vi "Timestamp_Compare.vi"() -> ()   [LabVIEW 2020]
panel:
  out "Camera Timestamp (UTC)":u64[](array[numeric])
  out "Camera Source Timestamp (UTC)":u64[](array[numeric])
  out "ENET First Timestamp Delta Difference":dbl format="%#_9g"
  out "CAN First Timestamp Delta Difference":dbl format="%#_9g"
  out "Camera First Timestamp Delta Difference":dbl[](array[numeric]) format="%#_9g"
  out "CAN Source Timestamp Delta":dbl format="%#_9f"
  out "ENET Source First Timestamp Delta":dbl format="%#_9f"
  in  "ENET Source T0 Time Stamp":timestamp=timestamp(3758873246.099163 s since 1904-01-01) format="%<%.6X\n%x>T"
  out "ENET First Timestamp Delta":dbl format="%#_9f"
  out "CAN First Timestamp Delta":dbl format="%#_9f"
  in  "ENET Receive First Time":timestamp=timestamp(3762227548.6655436 s since 1904-01-01) format="%<%.6X\n%x>T"
  in  "CAN Receive First Time":timestamp=timestamp(3762227536.6965528 s since 1904-01-01) format="%<%.6X\n%x>T"
  in  "CAN Source First Frame Relative Timestamp (s)":dbl=73.619141 format="%#_9g"
  in  "CAN Source T0 Time Stamp":timestamp=timestamp(3758873160.511 s since 1904-01-01)
  out "Camera Source First Timestamp Delta":dbl[](array[numeric]) format="%#_9f"
  out "Camera First Timestamp Delta":dbl[](array[numeric]) format="%#_9f"
  in  "Timestamp Compare Base Index":i32
  in  "Camera T0 TDMS":timestamp=timestamp(3762227502.1926026 s since 1904-01-01) format="%<%.6X\n%x>T"
  in  "Camera Source Timestamp Txt Path":path[](array[path])=[path "E:/Xiaomi_Source/RDMA_FVC0/time.txt", path "E:/Xiaomi_Source/RDMA_side0/time.txt"]
  in  "Source Timestamp from txt File":bool=TRUE
  out "error out":errorcluster
  in  "Camera Timestamp TDMS Path":path[](array[path])=[path "E:/Xiaomi_Test/4k_265_time.tdms", path "E:/Xiaomi_Test/2k_265_time.tdms"]
  in  "Skip First N Timestamp":i32=1
  in  "Camera Source_Timestamp (ns) type":T1(array[ring])
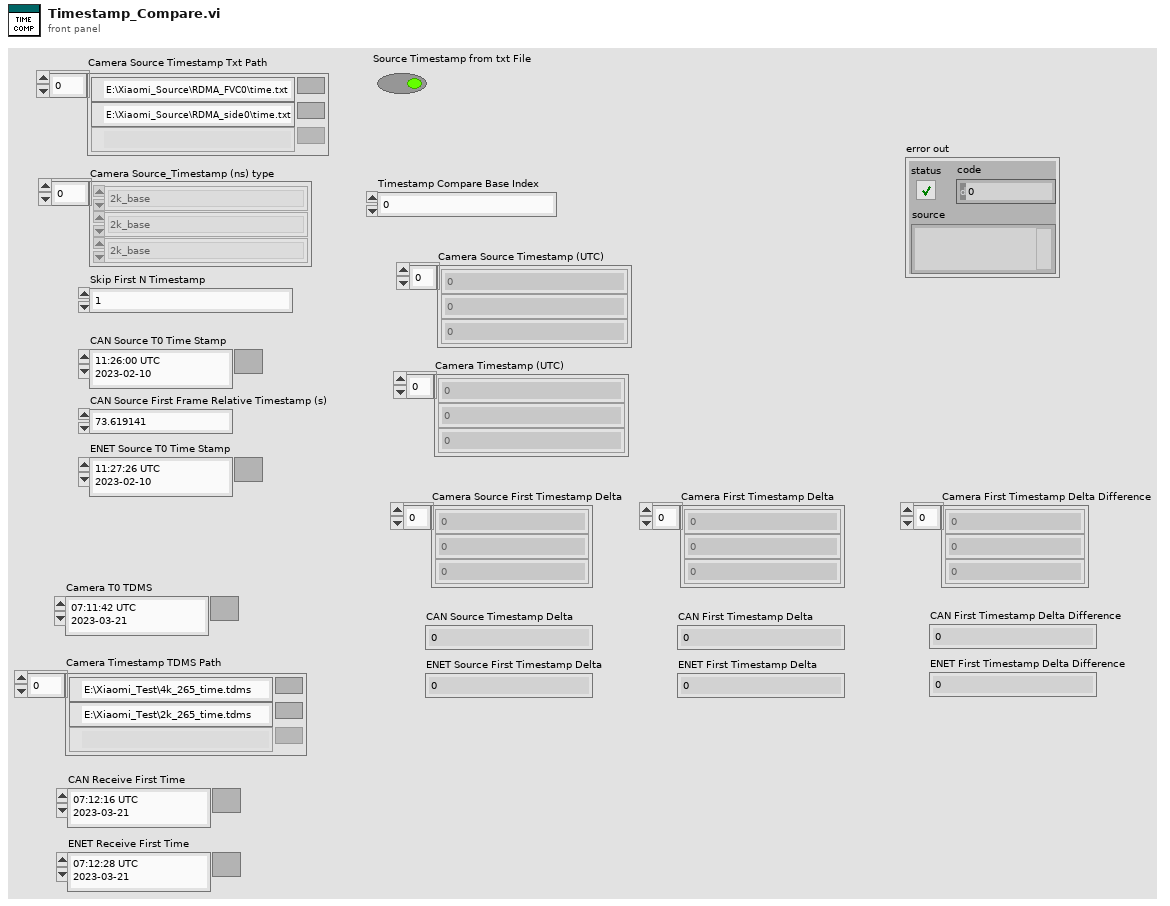
[diagram p1: front panel]
types:
  T1 = enum16{"2k_base", "2k_noise", "4k_base", "4k_noise"}[]
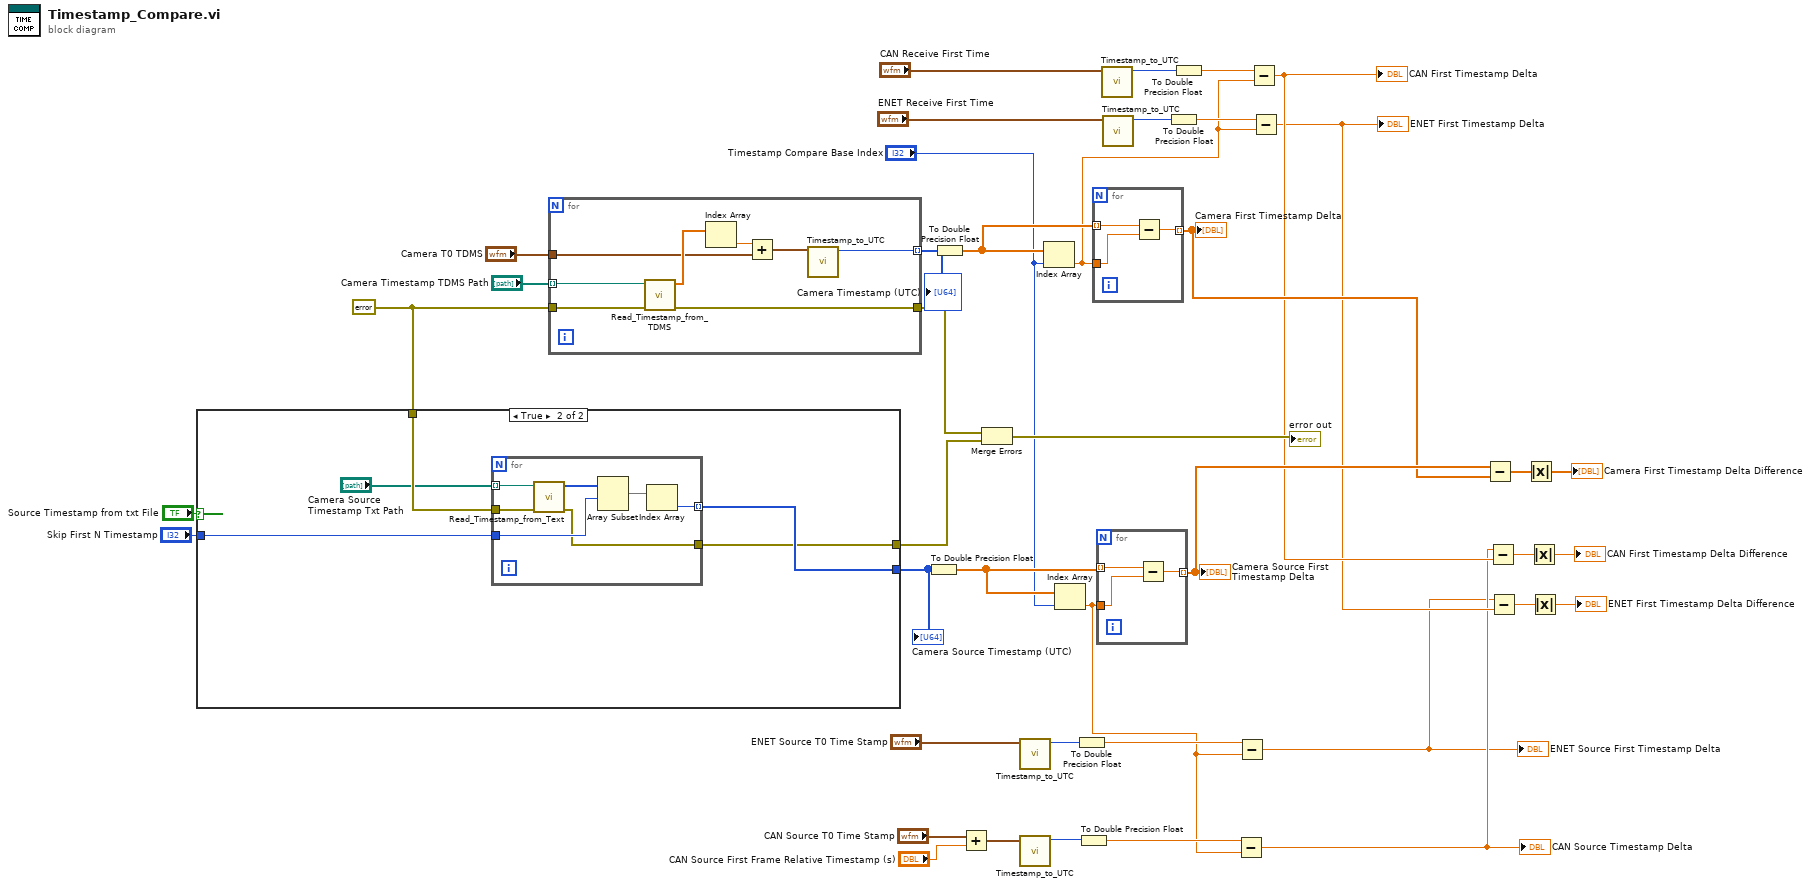
[diagram p0: block diagram]
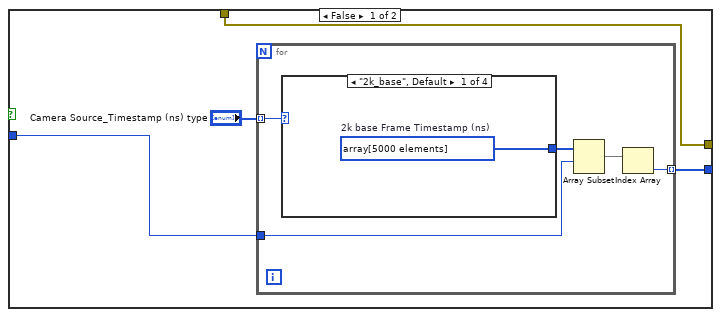
[diagram p2: hidden frame]
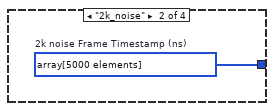
[diagram p3: hidden frame]
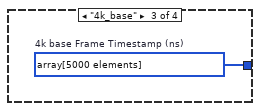
[diagram p4: hidden frame]
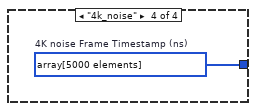
[diagram p5: hidden frame]
diagram:
  w40 = errorcluster {"status"=FALSE, "code"=0, "source"=""} ("error in (no error)")
  n1 = case shown="True" "Source Timestamp from txt File" {
    tunnel: w40 -> [w42 w59]
    tunnel: "Skip First N Timestamp" -> [w44 w57]
    tunnel: [w43 w56] -> w31
    tunnel: [w42 w55] -> w34
    frame False {
      n2 = for {
        tunnel: "Camera Source_Timestamp (ns) type" -> [w50] mode=indexing
        tunnel: w44 -> [w48]
        tunnel: [w46] -> w43 mode=indexing
        n3 = case shown="\"2k_base\", Default" w50 {
          tunnel: [w51 w52 w53 w54] -> w49
          frame "2k_base", Default {
            w51 = u64[] array[5000 elements]  # 2k base Frame Timestamp (ns)
          }
          frame "2k_noise" {
            w52 = u64[] array[5000 elements]  # 2k noise Frame Timestamp (ns)
          }
          frame "4k_base" {
            w53 = u64[] array[5000 elements]  # 4k base Frame Timestamp (ns)
          }
          frame "4k_noise" {
            w54 = u64[] array[5000 elements]  # 4K noise Frame Timestamp (ns)
          }
        }
        n4 = Array Subset(array=w49, index=w48) -> (w47:u64[])  [unwired: 1 in]
        n5 = Index Array(array=w47) -> (element=w46:u64)  [unwired: 1 in]
      }
    }
    frame True {
      n6 = for {
        tunnel: w59 -> [w66]
        tunnel: "Camera Source Timestamp Txt Path" -> [w65] mode=indexing
        tunnel: w57 -> [w62]
        tunnel: [w61] -> w56 mode=indexing
        tunnel: [w60] -> w55
        n7 = call "Read_Timestamp_from_Text.vi"("error in (no error)"=w66, "Txt File path"=w65) -> ("error out"=w60:errorcluster, "relative timestamp (ns)"=w63:u64[])  [unwired: 7 in, 1 out]
        n8 = Array Subset(array=w63, index=w62) -> (w64:u64[])  [unwired: 1 in]
        n9 = Index Array(array=w64) -> (element=w61:u64)  [unwired: 1 in]
      }
    }
  }
  "Camera Source Timestamp (UTC)" <- w31
  n10 = for {
    tunnel: w40 -> [w74]
    tunnel: [w73] -> w39
    tunnel: "Camera Timestamp TDMS Path" -> [w72] mode=indexing
    tunnel: "Camera T0 TDMS" -> [w69]
    tunnel: [w67] -> w33 mode=indexing
    n11 = call "Read_Timestamp_from_TDMS.vi"("error in (no error)"=w74, "TDMS File path"=w72) -> ("error out"=w73:errorcluster, "relative timestamp (s)"=w71:dbl[])  [unwired: 7 in, 1 out]
    n12 = Index Array(array=w71) -> (element=w70:dbl)  [unwired: 1 in]
    n13 = Add(x=w70, y=w69) -> (x+y=w68:timestamp)
    n14 = call "Timestamp_to_UTC.vi"("Timestamp"=w68) -> ("UTC Time"=w67:u64)  [unwired: 9 in, 1 out]
  }
  "Camera Timestamp (UTC)" <- w33
  n15 = To Double Precision Float(number=w31) -> (double precision float=w30:dbl[])
  n16 = To Double Precision Float(number=w33) -> (double precision float=w32:dbl[])
  n17 = Add(x="CAN Source T0 Time Stamp", y="CAN Source First Frame Relative Timestamp (s)") -> (x+y=w26:timestamp)
  n18 = Merge Errors(w39, w34) -> (→"error out":errorcluster)
  n19 = call "Timestamp_to_UTC.vi"("Timestamp"="ENET Source T0 Time Stamp") -> ("UTC Time"=w17:u64)  [unwired: 9 in, 1 out]
  n20 = call "Timestamp_to_UTC.vi"("Timestamp"=w26) -> ("UTC Time"=w16:u64)  [unwired: 9 in, 1 out]
  n21 = Index Array(array=w32, index="Timestamp Compare Base Index") -> (element=w19:dbl)
  n22 = Index Array(array=w30, index="Timestamp Compare Base Index") -> (element=w13:dbl)
  n23 = To Double Precision Float(number=w17) -> (double precision float=w15:dbl)
  n24 = To Double Precision Float(number=w16) -> (double precision float=w14:dbl)
  n25 = for {
    tunnel: w32 -> [w77] mode=indexing
    tunnel: w19 -> [w76]
    tunnel: [w75] -> w11 mode=indexing
    n26 = Subtract(x=w77, y=w76) -> (x-y=w75:dbl)
  }
  "Camera First Timestamp Delta" <- w11
  n27 = for {
    tunnel: w30 -> [w80] mode=indexing
    tunnel: w13 -> [w79]
    tunnel: [w78] -> w12 mode=indexing
    n28 = Subtract(x=w80, y=w79) -> (x-y=w78:dbl)
  }
  "Camera Source First Timestamp Delta" <- w12
  n29 = call "Timestamp_to_UTC.vi"("Timestamp"="CAN Receive First Time") -> ("UTC Time"=w23:u64)  [unwired: 9 in, 1 out]
  n30 = call "Timestamp_to_UTC.vi"("Timestamp"="ENET Receive First Time") -> ("UTC Time"=w21:u64)  [unwired: 9 in, 1 out]
  n31 = To Double Precision Float(number=w21) -> (double precision float=w20:dbl)
  n32 = To Double Precision Float(number=w23) -> (double precision float=w22:dbl)
  n33 = Subtract(x=w14, y=w13) -> (x-y=w4:dbl)
  "CAN Source Timestamp Delta" <- w4
  n34 = Subtract(x=w15, y=w13) -> (x-y=w3:dbl)
  "ENET Source First Timestamp Delta" <- w3
  n35 = Subtract(x=w22, y=w19) -> (x-y=w6:dbl)
  "CAN First Timestamp Delta" <- w6
  n36 = Subtract(x=w20, y=w19) -> (x-y=w5:dbl)
  "ENET First Timestamp Delta" <- w5
  n37 = Subtract(x=w12, y=w11) -> (x-y=w10:dbl[])
  n38 = Subtract(x=w4, y=w6) -> (x-y=w8:dbl)
  n39 = Subtract(x=w3, y=w5) -> (x-y=w7:dbl)
  n40 = Absolute Value(x=w10) -> (abs(x)=→"Camera First Timestamp Delta Difference":dbl[])
  n41 = Absolute Value(x=w8) -> (abs(x)=→"CAN First Timestamp Delta Difference":dbl)
  n42 = Absolute Value(x=w7) -> (abs(x)=→"ENET First Timestamp Delta Difference":dbl)
